vi "Compact pre metadata to one metadata.vi"(0 "appended array":T2[](array[typedef]), 5 "error in (no error)":errorcluster) -> (14 "Metadata":T1, 19 "error out":errorcluster)   [LabVIEW 2019, in "metadata.lvclass"]
uses:
  metadata.lvclass
  Metadata output --cluster.ctl
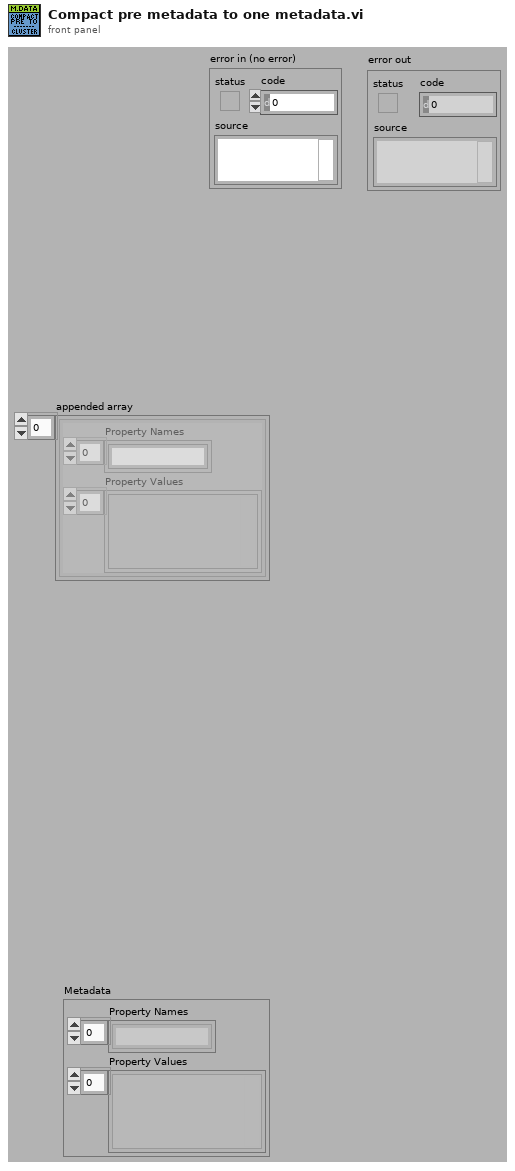
[diagram p1: front panel]
types:
  T1 = cluster{"Property Names":string[], "Property Values":variant[]}
  T2 = typedef "metadata.lvclass/Metadata output --cluster.ctl" = cluster{"Property Names":string[], "Property Values":variant[]}
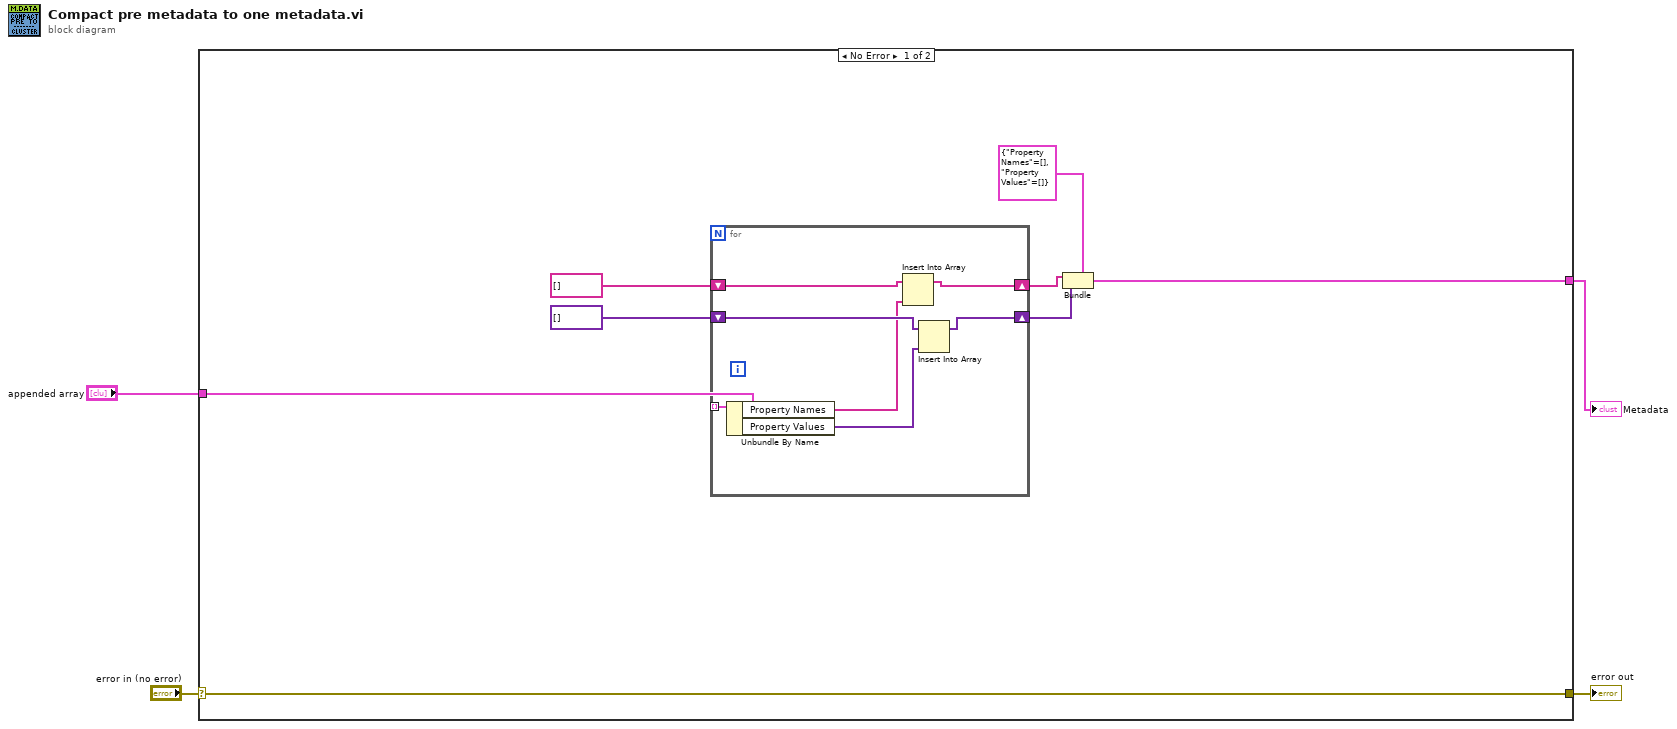
[diagram p0: block diagram]
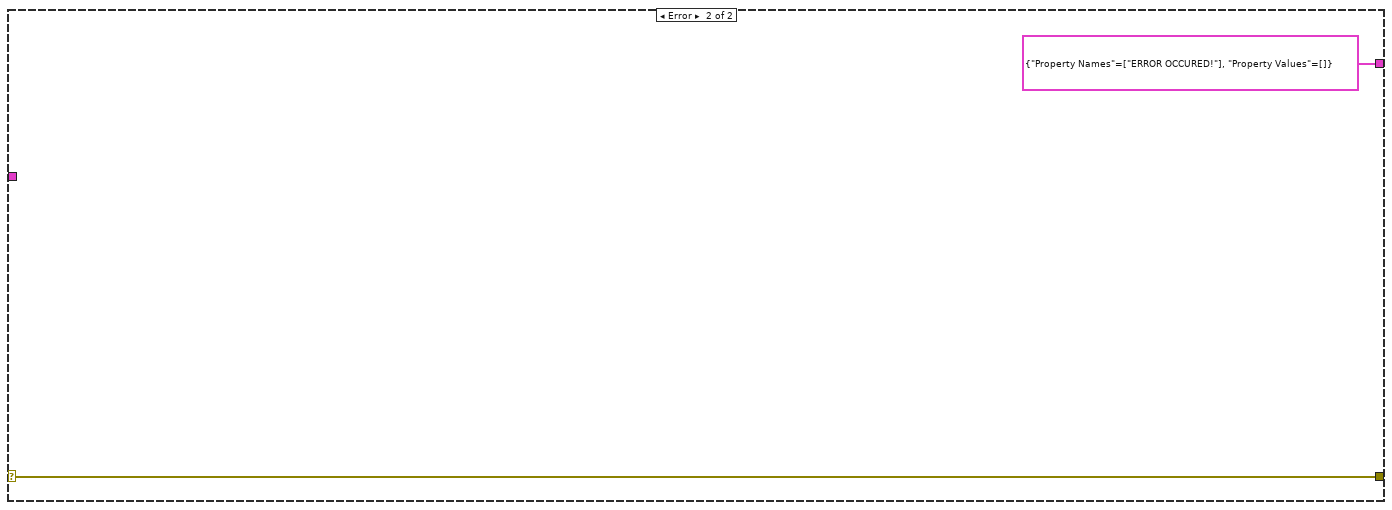
[diagram p2: hidden frame]
diagram:
  n1 = case shown="No Error" "error in (no error)" {
    selector: "error in (no error)" -> [w5 w21]
    tunnel: [w5 w21] -> w3
    tunnel: "appended array" -> [w12 _]
    tunnel: [w6 T1 {"Property Names"=["ERROR OCCURED!"], "Property Values"=[]} ("Metadata")] -> w1
    frame No Error {
      n2 = for {
        tunnel: w12 -> [w19] mode=indexing
        shift-right: [w13] -> w9
        shift-left: string[] [] ("Property Names") -> [w18]
        shift-right: [w14] -> w8
        shift-left: variant[] [] ("Property Values") -> [w17]
        n3 = Unbundle By Name(w19) -> ("Property Names"=w16:string[], "Property Values"=w15:variant[])
        n4 = Insert Into Array(array=w18, new element=w16) -> (w13:string[])  [unwired: 1 in]
        n5 = Insert Into Array(array=w17, new element=w15) -> (w14:variant[])  [unwired: 1 in]
      }
      n6 = Bundle(cluster=T1 {"Property Names"=[], "Property Values"=[]} ("Metadata"), "Property Names"=w9, "Property Values"=w8) -> (w6:T1)
    }
    frame Error {
    }
  }
  "error out" <- w3
  "Metadata" <- w1
